vi "deleteVariable.vi"(0 "HGF_DSCVarManager in":refnum<class "HGF_DSCVarManager.lvclass">, 2 "shared variable":refnum<k21>, 5 "error in (no error)":errorcluster) -> (14 "HGF_DSCVarManager out":refnum<class "HGF_DSCVarManager.lvclass">, 16 "not deleted?":bool, 19 "error out":errorcluster)   [LabVIEW 2012, in "HGF_DSC.lvlib" / "HGF_DSCVarManager.lvclass"]
uses:
  HGF_DSCVarManager.lvclass
  HGF_DSCVarManager.lvclass/HGF_DSCVarManager.ctl
  <vilib>/lvdsc/NI_DSC.lvlib
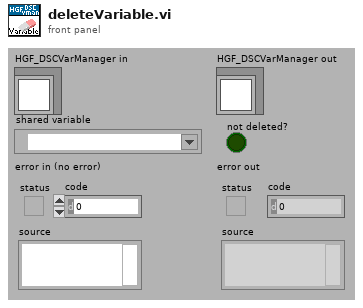
[diagram p1: front panel]
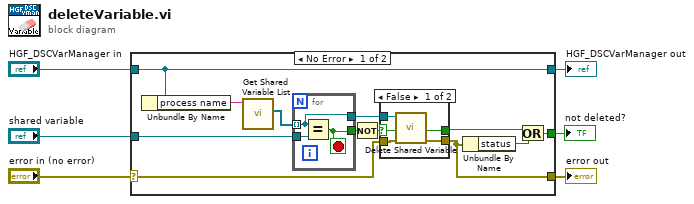
[diagram p0: block diagram]
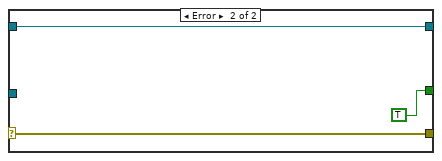
[diagram p3: hidden frame]
diagram:
  n1 = case shown="No Error" "error in (no error)" {
    selector: "error in (no error)" -> [w12 w30]
    tunnel: [w11 w30] -> w5
    tunnel: [w18 w29] -> w3
    tunnel: "HGF_DSCVarManager in" -> [w18 w29]
    tunnel: "shared variable" -> [w15 _]
    tunnel: [w7 TRUE] -> w1
    frame No Error {
      n2 = Unbundle By Name(w18) -> ("process name"=w17:string)
      n3 = call <vilib>:"Get Shared Variable List.vi"("process name"=w17) -> ("shared variables"=w16:refnum<k21>[])  [unwired: 1 in, 9 out]
      n4 = for {
        tunnel: w16 -> [w25] mode=indexing
        tunnel: w15 -> [w27]
        tunnel: [w26] -> w14
        tunnel: [w25] -> w13
        stop <- w26 stop-if-true
        n5 = Equal?(x=w25, y=w27) -> (x = y?=w26:bool)
      }
      n6 = Not(x=w14) -> (.not. x?=w10:bool)
      n7 = case shown="False" w10 {
        selector: w10 -> [w19 w23]
        tunnel: w13 -> [w22 _]
        tunnel: [w21 w24] -> w11
        tunnel: w12 -> [w20 w24]
        tunnel: [w19 w23] -> w8
        frame False {
          n8 = call <vilib>:"Delete Shared Variable.vi"("error in (no error)"=w20, "shared variable"=w22) -> ("error out"=w21:errorcluster)  [unwired: 9 out]
        }
        frame True {
        }
      }
      n9 = Unbundle By Name(w11) -> ("status"=w9:bool)
      n10 = Or(x=w8, y=w9) -> (x .or. y?=w7:bool)
    }
    frame Error {
    }
  }
  "error out" <- w5
  "HGF_DSCVarManager out" <- w3
  "not deleted?" <- w1
